vi "Standard Engine.vi"(8 "error in":errorcluster, 11 "Engine Process Init Data":T1) -> (0 "error out":errorcluster)   [LabVIEW 2013, in "Standard Engine Runtime.lvclass"]
doc: "This VI is a process that executes modules and has an API for transitioning through its state machine. Once it is initialized and running, it calls an array of module input methods, followed by an array of module process methods, followed by an array of module output methods, and then does any necessary error handling and bookkeeping."
uses:
  Standard Engine Runtime.lvclass
  Engine Process Init Data.ctl
  Commands.ctl
  Engine Config Data.ctl
  Configuration/Standard Engine Configuration.lvclass
  <vilib>/NI/Tag Bus Module Framework/runtime/TBM module execution interface.lvclass
  <vilib>/NI/Tag Bus Module Framework/module configuration/TBM module configuration.lvclass
  <vilib>/NI/Module Execution Interface/Engine Runtime/Execution States.ctl
  Engine Data.ctl
  Configuration/Loop Info.ctl
  <vilib>/NI/Tag Bus/table/data table.ctl
  Module Execution Info.ctl
  Data Table with Transfer Spec.ctl
  <vilib>/NI/Tag Bus/table/transfer specification.ctl
  <vilib>/NI/Tag Bus/tag/Data Type.ctl
  Configuration/Module Decimation.ctl
  Configuration/Module Error Configuration.ctl
  Configuration/Error Actions By Category.ctl
  <vilib>/NI/Tag Bus Module Framework/runtime/error classification.ctl
  Configuration/Error Actions.ctl
  <vilib>/NI/Module Timing Source/timing source/TBM timing source.lvclass
  Configuration/timing policy.ctl
  async execution info.ctl
  asynchronous process data.ctl
  async command notification.ctl
  <vilib>/NI/Tag Bus Module Framework/runtime/execution settings.ctl
  async error info.ctl
  status reporting data.ctl
  module status reporting.ctl
  <vilib>/Platform/TimedLoop/XDataNode/timing_clust.ctl
  <vilib>/Platform/TimedLoop/XDataNode/nitl_modes.ctl
  <vilib>/Platform/TimedLoop/XDataNode/wakeup.ctl
  <vilib>/NI/Module Timing Source/timing source/TBM timing source.lvclass/TBM timing source.ctl
  <vilib>/NI/Tag Bus/table/transfer table data.vi
  Module Execution Decimation.vi
  Error Handler.vi
  <vilib>/NI/Tag Bus/table/write data element.vi
  <vilib>/NI/Tag Bus/table/data polymorphs/write one/write Boolean.vi
  <vilib>/NI/Tag Bus/table/data polymorphs/write one/write U32.vi
  <vilib>/NI/Tag Bus/table/data polymorphs/write one/write U64.vi
  <vilib>/NI/Tag Bus/table/data polymorphs/write one/write I32.vi
  Delete Module Index.vi
  <vilib>/platform/TimedLoop/XDataNode/XDataNode.xnode
  <vilib>/NI/Module Execution Interface/Engine Runtime/Engine Runtime Interface.lvclass
  <vilib>/NI/Tag Bus/table/data table.lvlib
  <vilib>/NI/Tag Bus/tag/tag descriptor.lvclass
  <vilib>/Platform/TimedLoop/XDataNode/XDNodeRunTimeDep.lvlib
panel:
  out "iterations":i32
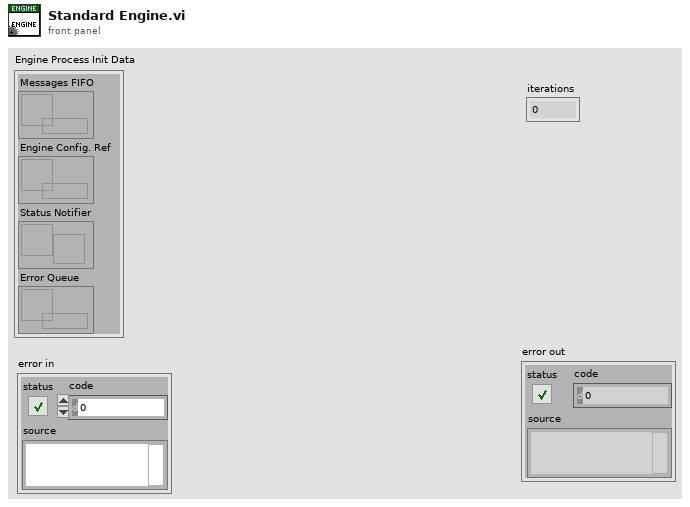
[diagram p1: front panel]
types:
  T1 = typedef "Standard Engine Runtime.lvclass/Engine Process Init Data.ctl" = cluster{"Messages FIFO":refnum<k33>, "Engine Config. Ref":refnum<data-value>, "Status Notifier":refnum<notifier>, "Error Queue":refnum<queue>}
  T2 = typedef "Standard Engine Runtime.lvclass/Engine Data.ctl" = cluster{"Loop Info":T3, "Main Tag Data":T4, "Module Info":T5, "engine timing source":refnum<class "TBM timing source.lvclass">, "timing policy":T14, "async execution info":T15, "status reporting":T18}
  T3 = typedef "Standard Engine Configuration.lvclass/Loop Info.ctl" = cluster{"Processor":i32, "Priority":i32}
  T4 = typedef "tag bus.lvlib/data table.lvlib/data table.ctl" = cluster{"Double":dbl[], "Single":sgl[], "I64":i64[], "I32":i32[], "I16":i16[], "I8":i8[], "U64":u64[], "U32":u32[], "U16":u16[], "U8":u8[], "Boolean":bool[], "String":string[], "Array of Double":cluster{"DBL Array":dbl[]}[], "Array of Single":cluster{"SGL Array":sgl[]}[], "Array of I64":cluster{"I64 Array":i64[]}[], "Array of I32":cluster{"I32 Array":i32[]}[], "Array of I16":cluster{"I16 Array":i16[]}[], "Array of I8":cluster{"I8 Array":i8[]}[], "Array of U64":cluster{"U64 Array":u64[]}[], "Array of U32":cluster{"U32 Array":u32[]}[], "Array of U16":cluster{"U16 Array":u16[]}[], "Array of U8":cluster{"U8 Array":u8[]}[], "Array of Boolean":cluster{"Boolean Array":bool[]}[], "Array of String":cluster{"String Array":string[]}[]}
  T5 = typedef "Standard Engine Runtime.lvclass/Module Execution Info.ctl" = cluster{"Tag Bus Modules":refnum<class "TBM module execution interface.lvclass">[], "Execute?":bool[], "Input Method Indices":i32[], "Process Method Indices":i32[], "Output Method Indices":i32[], "Input Transfer Specifications":T6[], "Parameter Transfer Specifications":T6[], "Result Transfer Specifications":T6[], "Output Transfer Specifications":T6[], "Module Errors":errorcluster[], "Module Decimation":T9[], "Module Decimation Indices":i32[], "Error Queue":refnum<queue>, "Module Error Configuration":T10[], "Module Errors (n-1)":errorcluster[]}
  T6 = typedef "Standard Engine Runtime.lvclass/Data Table with Transfer Spec.ctl" = cluster{"Data Table":T4, "Transfer Specification":T7[]}
  T7 = typedef "tag bus.lvlib/data table.lvlib/transfer specification.ctl" = cluster{"data type":T8, "sink indices":i32[], "source indices":i32[]}
  T8 = typedef "tag bus.lvlib/tag descriptor.lvclass/Data Type.ctl" = enum16{"Double", "Single", "I64", "I32", "I16", "I8", "U64", "U32", "U16", "U8", "Boolean", "String", "Array of Double", "Array of Single", "Array of I64", "Array of I32", "Array of I16", "Array of I8", "Array of U64", "Array of U32", "Array of U16", "Array of U8", "Array of Boolean", "Array of String"}
  T9 = typedef "Standard Engine Configuration.lvclass/Module Decimation.ctl" = cluster{"Decimation":u16, "Offset":u16}
  T10 = typedef "Standard Engine Configuration.lvclass/Module Error Configuration.ctl" = cluster{"Module Error Configuration":T11[]}
  T11 = typedef "Standard Engine Configuration.lvclass/Error Actions By Category.ctl" = cluster{"error classification":T12, "Error Actions":T13[]}
  T12 = typedef "TBM module execution interface.lvclass/error classification.ctl" = enum16{"unknown", "none", "trivial", "recoverable", "critical"}
  T13 = typedef "Standard Engine Configuration.lvclass/Error Actions.ctl" = enum16{"Clear", "Notify", "Stop Component", "Stop Engine", "Safe State", "Attempt Recovery"}
  T14 = typedef "Standard Engine Configuration.lvclass/timing policy.ctl" = enum16{"strict determinism", "nonblocking", "nondeterministic inline"}
  T15 = typedef "Standard Engine Runtime.lvclass/async execution info.ctl" = cluster{"Tag Bus Modules":T16[], "Execute?":bool[], "Input Method Indices":i32[], "Process Method Indices":i32[], "Output Method Indices":i32[], "Input Transfer Specifications":T6[], "Parameter Transfer Specifications":T6[], "Result Transfer Specifications":T6[], "Output Transfer Specifications":T6[], "Module Errors":errorcluster[], "Module Decimation":T9[], "Module Decimation Indices":i32[], "Error Queue":refnum<queue>, "Module Error Configuration":T10[], "comm errors":errorcluster[]}
  T16 = typedef "Standard Engine Runtime.lvclass/asynchronous process data.ctl" = cluster{"thread reference":refnum<vi>, "cmd notification":refnum<k33>, "execution period (ms)":i32, "input from component":refnum<queue>, "input to component":refnum<queue>, "output from component":refnum<queue>, "output to component":refnum<queue>, "process input from component":refnum<queue>, "process input to component":refnum<queue>, "process result from component":refnum<queue>, "process result to component":refnum<queue>, "execution settings":T17, "error fifo":refnum<k33>}
  T17 = typedef "TBM module execution interface.lvclass/execution settings.ctl" = cluster{"reads inputs":bool, "processes data":bool, "writes outputs":bool}
  T18 = typedef "Standard Engine Runtime.lvclass/status reporting data.ctl" = cluster{"late index (bool)":i32, "late count (U32)":i32, "current dt ns(U64)":i32, "synchronous modules":T19[], "asynchronous modules":T19[]}
  T19 = typedef "Standard Engine Runtime.lvclass/module status reporting.ctl" = cluster{"module index":i32, "error tag (I32)":i32}
  T20 = typedef "Engine Runtime Interface.lvclass/Execution States.ctl" = enum16{"Initializing", "Paused (Initialized)", "Running", "Set Safe Outputs", "Uninitializing", "Stopped (Uninitialized)", "Error (Uninitialized)", "Safe State (Uninitialized)", "Closed"}
  T21 = typedef "Standard Engine Runtime.lvclass/Commands.ctl" = enum16{"Initialize", "Start", "Pause", "Safe State", "Normal", "Stop", "Shutdown"}
  T22 = typedef "XDNodeRunTimeDep.lvlib/timing_clust.ctl" = cluster{"Expected End [f-1]":u64, "Actual End [f-1]":u64, "Finished Late? [f-1]":bool, "Expected End [i-1]":u64, "Actual End [i-1]":u64, "Finished Late? [i-1]":bool, "Expected Start [i]":u64, "Actual Start [i]":u64, "Expected Start [f]":u64, "Actual Start [f]":u64, "Source Name":string, "Structure Name":string, "Period":i64, "Deadline":i64, "Offset":i64, "Start":i64, "Priority":i32, "Timeout":i32, "Mode":T23, "Wakeup Reason":T24, "Error":errorcluster, "Source Type":string, "Secondary Source Type":string, "Global End Time":u64, "Global Start Time":u64, "Frame Duration":u64, "Iteration Duration":u64, "Assigned CPU":i32, "I/O Scan Engine Mode":u32}
  T23 = typedef "XDNodeRunTimeDep.lvlib/nitl_modes.ctl" = enum32{"No Change", "Process missed periods, maintain original phase", "Discard missed periods, maintain original phase", "Process missed periods, ignore original phase", "Discard missed periods, ignore original phase"}
  T24 = typedef "XDNodeRunTimeDep.lvlib/wakeup.ctl" = enum32{"Normal", "Aborted", "Asynchronous wakeup", "Timing source error", "Timed loop error", "Timeout"}
  T25 = typedef "Standard Engine Runtime.lvclass/Engine Config Data.ctl" = cluster{"Engine Configuration":refnum<class "Standard Engine Configuration.lvclass">, "Modules":refnum<class "TBM module execution interface.lvclass">[], "Module Configurations":refnum<class "TBM module configuration.lvclass">[]}
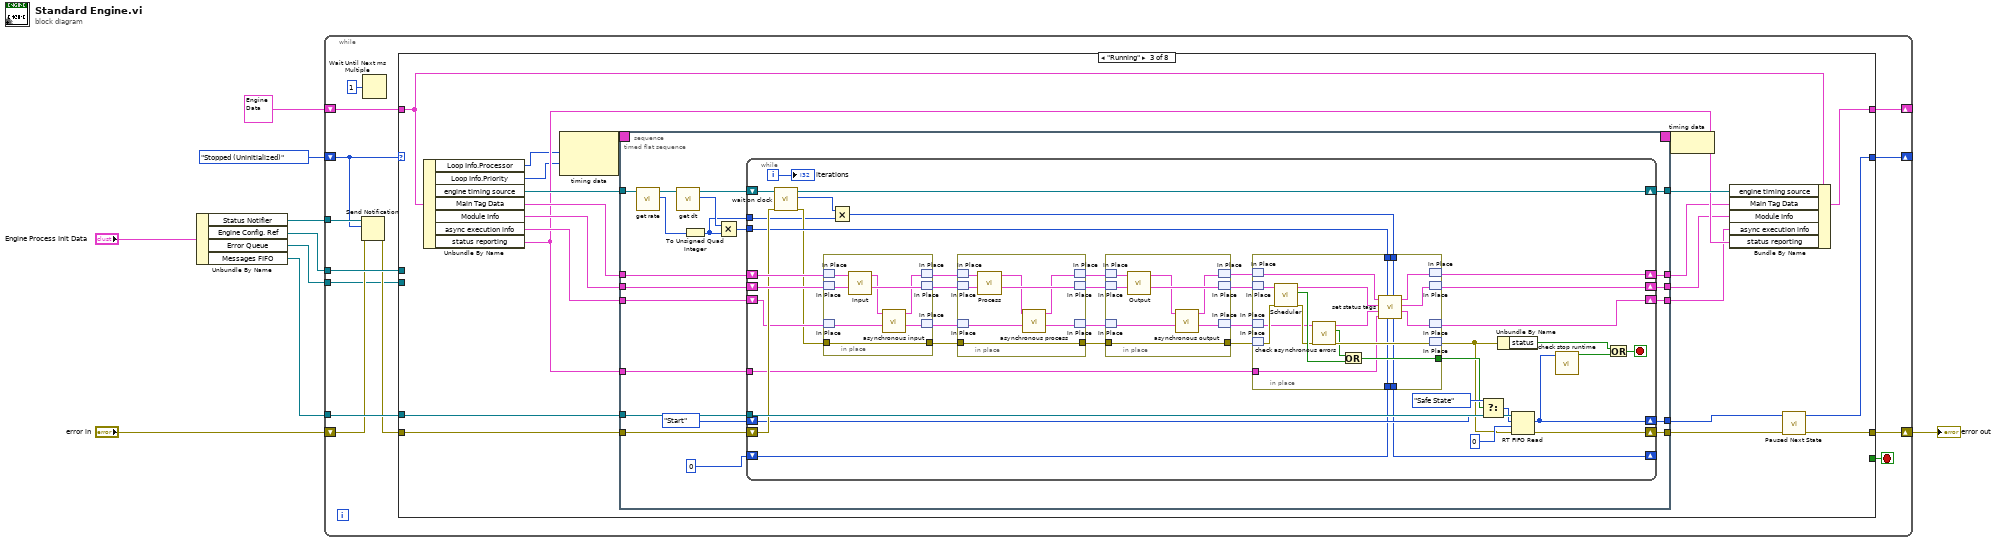
[diagram p0: block diagram]
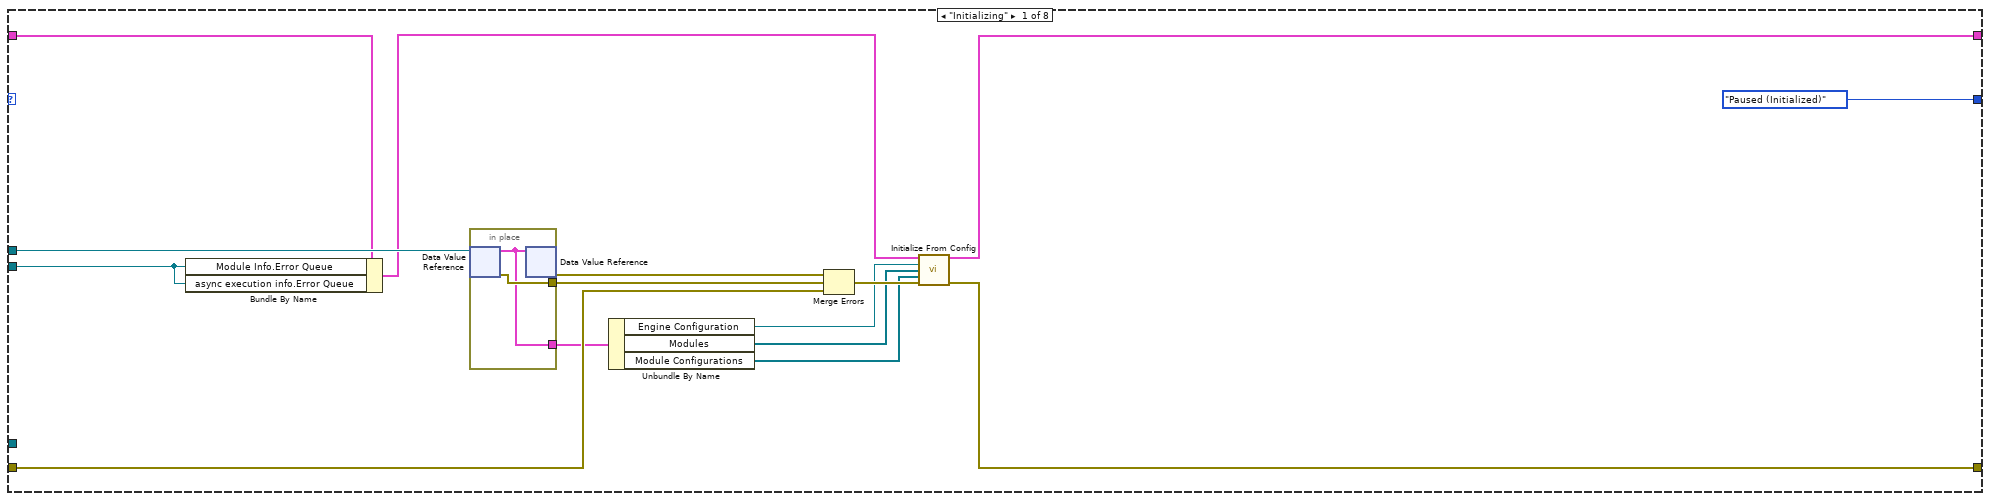
[diagram p2: hidden frame]
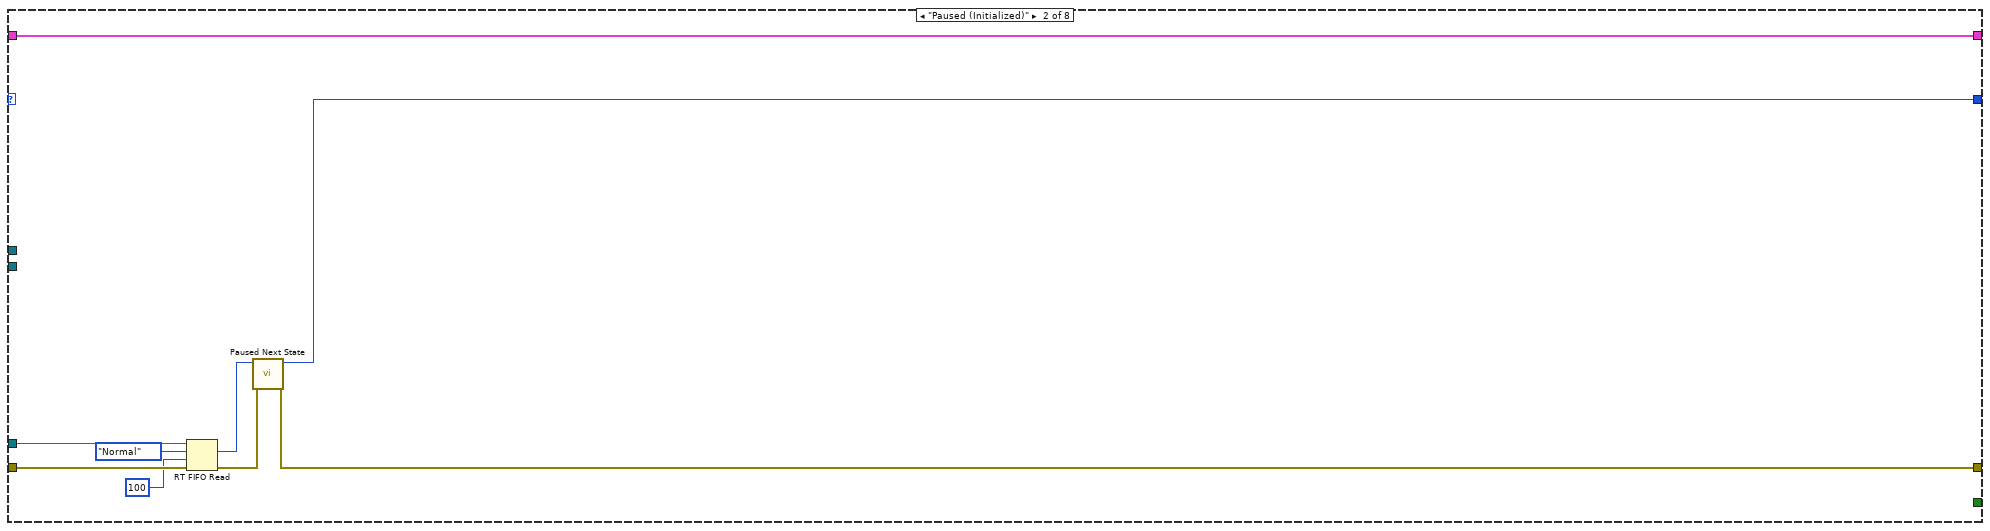
[diagram p3: hidden frame]
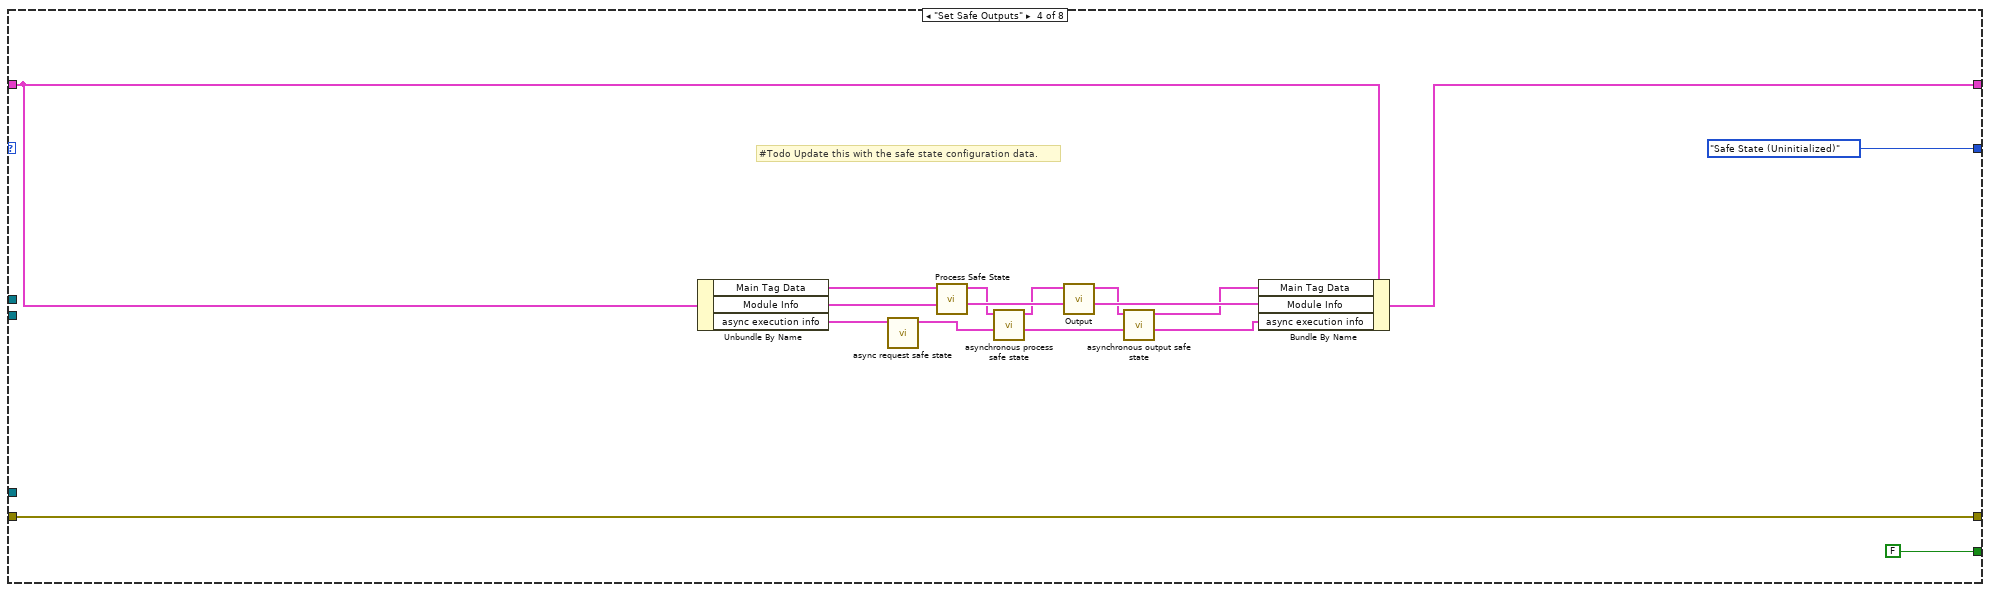
[diagram p4: hidden frame]
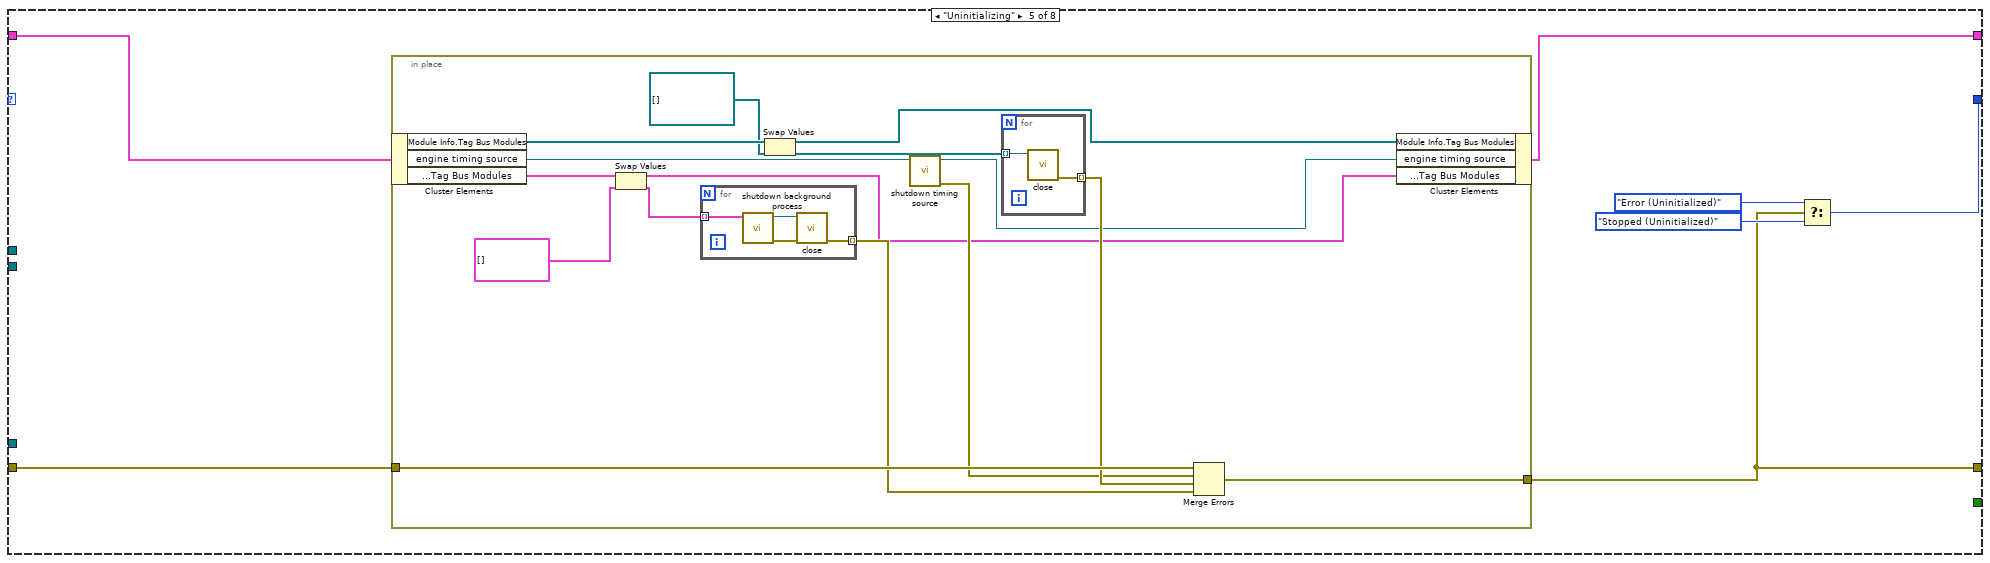
[diagram p5: hidden frame]
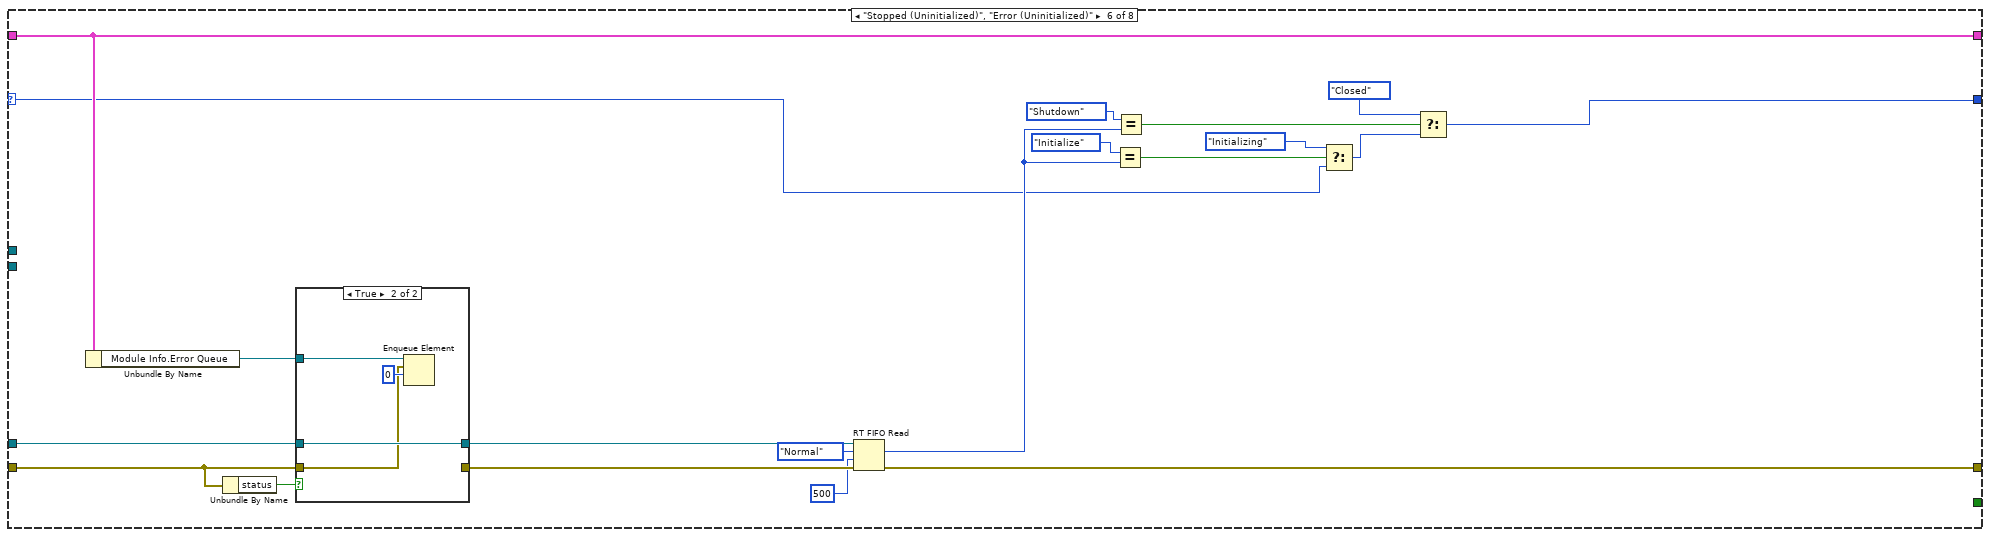
[diagram p6: hidden frame]
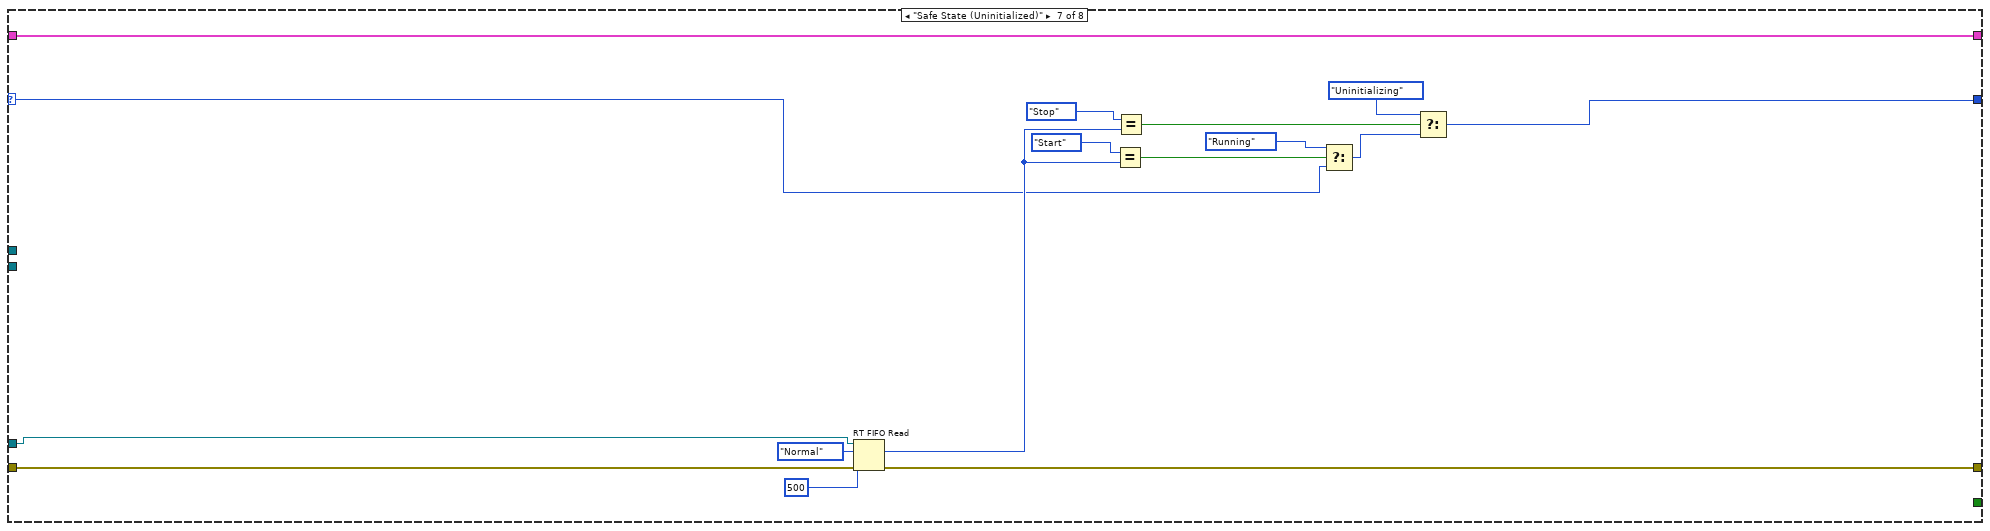
[diagram p8: hidden frame]
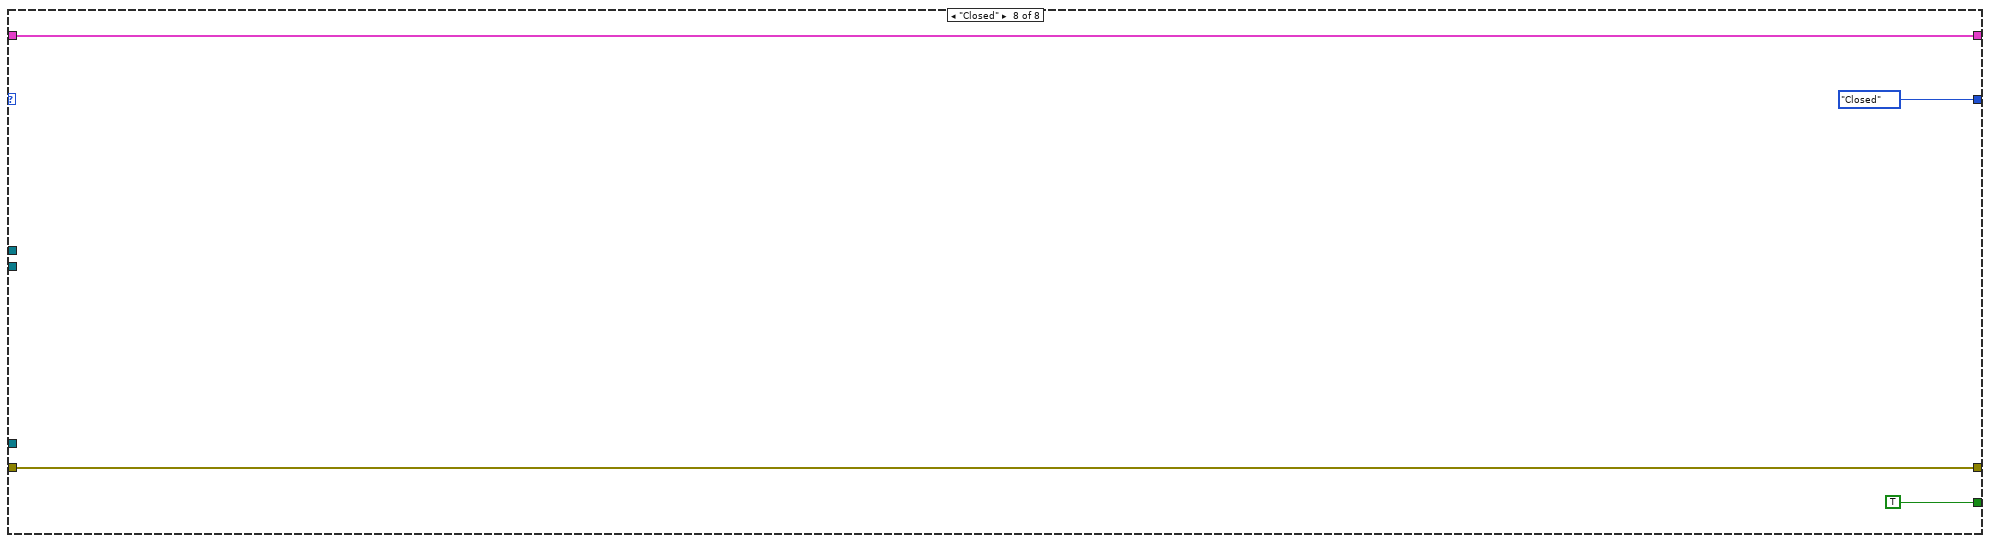
[diagram p9: hidden frame]
diagram:
  n1 = Unbundle By Name("Engine Process Init Data") -> ("Status Notifier"=w7:refnum<notifier>, "Engine Config. Ref"=w6:refnum<data-value>, "Error Queue"=w3:refnum<queue>, "Messages FIFO"=w5:refnum<k33>)
  n2 = while {
    shift-right: [w19] -> _
    shift-left: Execution_States."Stopped (Uninitialized)" ("States") -> [w14]
    shift-right: [w20] -> _
    shift-left: T2 {"Loop Info"={"Processor"=-2, "Priority"=0}, "Main Tag Data"={"Double"=[], "Single"=[], "I64"=[], "I32"=[], "I16"=[], "I8"=[], "U64"=[], "U32"=[], "U16"=[], "U8"=[], "Boolean"=[], "String"=[], "Array of Double"=[], "Array of Single"=[], "Array of I64"=[], "Array of I32"=[], "Array of I16"=[], "Array of I8"=[], "Array of U64"=[], "Array of U32"=[], "Array of U16"=[], "Array of U8"=[], "Array of Boolean"=[], "Array of String"=[]}, "Module Info"={"Tag Bus Modules"=[], "Execute?"=[], "Input Method Indices"=[], "Process Method Indices"=[], "Output Method Indices"=[], "Input Transfer Specifications"=[], "Parameter Transfer Specifications"=[], "Result Transfer Specifications"=[], "Output Transfer Specifications"=[], "Module Errors"=[], "Module Decimation"=[], "Module Decimation Indices"=[], "Error Queue"=refnum, "Module Error Configuration"=[], "Module Errors (n-1)"=[]}, "engine timing source"=refnum, "timing policy"=enum."nonblocking", "async execution info"={"Tag Bus Modules"=[], "Execute?"=[], "Input Method Indices"=[], "Process Method Indices"=[], "Output Method Indices"=[], "Input Transfer Specifications"=[], "Parameter Transfer Specifications"=[], "Result Transfer Specifications"=[], "Output Transfer Specifications"=[], "Module Errors"=[], "Module Decimation"=[], "Module Decimation Indices"=[], "Error Queue"=refnum, "Module Error Configuration"=[], "comm errors"=[]}, "status reporting"={"late index (bool)"=0, "late count (U32)"=0, "current dt ns(U64)"=0, "synchronous modules"=[], "asynchronous modules"=[]}} ("Engine Data Out") -> [w22]
    shift-right: [w21] -> w8
    shift-left: "error in" -> [w13]
    tunnel: w5 -> [w18]
    tunnel: w6 -> [w16]
    tunnel: w7 -> [w15]
    tunnel: w3 -> [w11]
    stop <- w17 stop-if-true
    n3 = Send Notification(notification=w14, notifier=w15, error in (no error)=w13) -> (error out=w12:errorcluster)  [unwired: 1 out]
    n4 = Wait Until Next ms Multiple(millisecond multiple=u32 1) -> ()  [unwired: 1 out]
    n5 = case shown="\"Running\"" w14 {
      selector: w14 -> [_ _ _ _ _ w245 w269 _]
      tunnel: w22 -> [w26 w48 w67 w208 w214 w247 w270 w284]
      tunnel: w12 -> [w34 w47 w53 w212 w216 w241 w272 w286]
      tunnel: [w24 w42 w65 w212 w215 w256 w279 w286] -> w21
      tunnel: [w32 w48 w66 w209 w213 w247 w270 w284] -> w20
      tunnel: [Execution_States."Paused (Initialized)" ("States") w46 w68 Execution_States."Safe State (Uninitialized)" ("States") w217 w257 w280 Execution_States."Closed" ("States")] -> w19
      tunnel: w18 -> [_ w41 w69 _ _ w249 w271 _]
      tunnel: [_ _ _ FALSE _ _ _ TRUE] -> w17
      tunnel: w16 -> [w29 _ _ _ _ _ _ _]
      tunnel: w11 -> [w23 _ _ _ _ _ _ _]
      frame "Initializing" {
        n6 = Bundle By Name(cluster=w26, "Module Info.Error Queue"=w23, "async execution info.Error Queue"=w23) -> (w25:T2)
        n7 = in-place {
          in-place-border: [w39] -> w35
          in-place-border: [w38] -> w33
          n8 = in-place-dvr #1(w29) -> (w38:T25, w39:errorcluster)
          n9 = in-place-dvr #1(w38) -> (w36:errorcluster)  [unwired: 1 out]
        }
        n10 = Unbundle By Name(w33) -> ("Engine Configuration"=w30:refnum<class "Standard Engine Configuration.lvclass">, "Modules"=w28:refnum<class "TBM module execution interface.lvclass">[], "Module Configurations"=w27:refnum<class "TBM module configuration.lvclass">[])
        n11 = Merge Errors(w36, w35, w34) -> (w31:errorcluster)
        n12 = call "Initialize From Config.vi"("Engine Data"=w25, "Engine Configuration"=w30, "Modules"=w28, "Module Configurations"=w27, "error in"=w31) -> ("Engine Data Out"=w32:T2, "error out"=w24:errorcluster)  [unwired: 9 in]
      }
      frame "Paused (Initialized)" {
        n13 = RT FIFO Read(0:w41, 1:Commands."Normal" ("Commands"), 2:100 ("timeout in ms (0)"), 3:w47) -> (9:w45:T21, 11:w44:errorcluster)  [unwired: 3 out]
        n14 = call "Paused Next State.vi"("error in"=w44, "Command"=w45) -> ("error out"=w42:errorcluster, "State"=w46:T20)  [unwired: 8 in]
      }
      frame "Running" {
        n15 = Unbundle By Name(w67) -> ("Loop Info.Processor"=w50:i32, "Loop Info.Priority"=w49:i32, "engine timing source"=w62:refnum<class "TBM timing source.lvclass">, "Main Tag Data"=w61:T4, "Module Info"=w60:T5, "async execution info"=w59:T15, "status reporting"=w57:T18)
        n16 = node-c288(w50, w49) -> (w52:T22)
        n17 = timed-sequence {
          timing: w52 -> [_]
          timing-out: [_] -> w51
          tunnel: w69 -> [w82]
          tunnel: [w81] -> w64
          tunnel: [w80] -> w63
          tunnel: w62 -> [w70]
          tunnel: w61 -> [w79]
          tunnel: w60 -> [w78]
          tunnel: w59 -> [w77]
          tunnel: [w76] -> w58
          tunnel: w57 -> [w75]
          tunnel: [w74] -> w56
          tunnel: [w73] -> w55
          tunnel: [w72] -> w54
          tunnel: w53 -> [w71]
          n18 = timed-flat-sequence {
            tunnel: w82 -> [w103]
            tunnel: [w102] -> w81
            tunnel: [w101] -> w80
            tunnel: w79 -> [w100]
            tunnel: w78 -> [w99]
            tunnel: w77 -> [w98]
            tunnel: [w97] -> w76
            tunnel: w75 -> [w96]
            tunnel: [w95] -> w74
            tunnel: [w94] -> w73
            tunnel: [w93] -> w72
            tunnel: w71 -> [w89]
            tunnel: w70 -> [w88]
            n19 = call-dynamic "get rate.vi"("timing source in"=w88) -> ("period (ns)"=w84:i64, "timing source out"=w87:refnum<class "TBM timing source.lvclass">)  [unwired: 8 in, 1 out]
            n20 = call <vilib>:"get dt.vi"("timing source in"=w87) -> ("dt"=w85:u32, "timing source out"=w91:refnum<class "TBM timing source.lvclass">)  [unwired: 9 in]
            n21 = To Unsigned Quad Integer(1:w84) -> (0:w83:u64)
            n22 = Multiply(x=w85, y=w83) -> (x*y=w86:u64)
            n23 = while {
              tunnel: w103 -> [w135]
              shift-right: [w137] -> w102
              shift-left: Commands."Start" ("Commands") -> [w123]
              shift-right: [w117] -> w95
              shift-left: w100 -> [w144]
              shift-right: [w138] -> w94
              shift-left: w99 -> [w143]
              shift-right: [w134] -> w101
              shift-left: w89 -> [w130]
              shift-right: [w129] -> w97
              shift-left: w91 -> [w131]
              tunnel: w86 -> [w116]
              shift-right: [w124] -> w93
              shift-left: w98 -> [w128]
              tunnel: w96 -> [w115]
              shift-right: [w114] -> _
              shift-left: u32 0 ("late count out") -> [w113]
              tunnel: w83 -> [w108]
              i -> [w133]
              stop <- w105 stop-if-true
              n24 = call-dynamic "wait on clock.vi"("error in"=w130, "timing source in"=w131) -> ("error out"=w112:errorcluster, "ticks since last call"=w107:u32, "timing source out"=w129:refnum<class "TBM timing source.lvclass">)  [unwired: 7 in]
              n25 = in-place {
                in-place-border: w112 -> [w184]
                in-place-border: [w184] -> w109
                n26 = in-place-match #2(w144) -> (w183:T4)
                n27 = in-place-match #3(w143) -> (w188:T5)
                n28 = in-place-match #4(w128) -> (w186:T15)
                n29 = call "Input.vi"("Module Info In"=w188, "Engine Tags In"=w183) -> ("Module Info Out"=w187:T5, "Engine Tags Out"=w182:T4)  [unwired: 8 in]
                n30 = call "asynchronous input.vi"("Module Info In"=w186, "Engine Tags In"=w182) -> ("Module Info Out"=w185:T15, "Engine Tags Out"=w181:T4)  [unwired: 8 in]
                n31 = in-place-match #2(w181) -> (w142:T4)
                n32 = in-place-match #3(w187) -> (w141:T5)
                n33 = in-place-match #4(w185) -> (w127:T15)
              }
              n34 = Multiply(x=w107, y=w108) -> (x*y=w106:u64)
              n35 = in-place {
                in-place-border: [w173] -> w110
                in-place-border: w109 -> [w173]
                n36 = in-place-match #5(w142) -> (w179:T4)
                n37 = in-place-match #6(w141) -> (w180:T5)
                n38 = in-place-match #7(w127) -> (w177:T15)
                n39 = call "Process.vi"("Module Info In"=w180, "Engine Tags In"=w179) -> ("Module Info Out"=w178:T5, "Engine Tags Out"=w176:T4)  [unwired: 8 in]
                n40 = call "asynchronous process.vi"("Module Info In"=w177, "Engine Tags In"=w176) -> ("Module Info Out"=w175:T15, "Engine Tags Out"=w174:T4)  [unwired: 8 in]
                n41 = in-place-match #5(w174) -> (w132:T4)
                n42 = in-place-match #6(w178) -> (w140:T5)
                n43 = in-place-match #7(w175) -> (w126:T15)
              }
              n44 = in-place {
                in-place-border: [w165] -> w111
                in-place-border: w110 -> [w165]
                n45 = in-place-match #8(w132) -> (w172:T4)
                n46 = in-place-match #9(w140) -> (w171:T5)
                n47 = in-place-match #10(w126) -> (w169:T15)
                n48 = call "Output.vi"("Module Info In"=w171, "Engine Tags In"=w172) -> ("Module Info Out"=w170:T5, "Engine Tags Out"=w167:T4)  [unwired: 8 in]
                n49 = call "asynchronous output.vi"("Module Info In"=w169, "Engine Tags In"=w167) -> ("Module Info Out"=w168:T15, "Engine Tags Out"=w166:T4)  [unwired: 8 in]
                n50 = in-place-match #8(w166) -> (w118:T4)
                n51 = in-place-match #9(w170) -> (w139:T5)
                n52 = in-place-match #10(w168) -> (w125:T15)
              }
              n53 = in-place {
                in-place-border: [w160] -> w120
                in-place-border: w116 -> [w147]
                in-place-border: w106 -> [w146]
                in-place-border: w115 -> [w148]
                in-place-border: [w150] -> w114
                in-place-border: w113 -> [w149]
                n54 = in-place-match #11(w118) -> (w156:T4)
                n55 = in-place-match #12(w139) -> (w157:T5)
                n56 = in-place-match #13(w125) -> (w158:T15)
                n57 = in-place-match #14(w111) -> (w164:errorcluster)
                n58 = call "Scheduler.vi"("error in"=w164, "Module Info In"=w157) -> ("error out"=w162:errorcluster, "Safe State?"=w163:bool, "Module Info Out"=w155:T5)  [unwired: 7 in]
                n59 = call "check asynchronous errors.vi"("error in"=w162, "Module Info In"=w158) -> ("error out"=w161:errorcluster, "safe state?"=w159:bool, "Module Info Out"=w152:T15)  [unwired: 7 in]
                n60 = Or(x=w159, y=w163) -> (x .or. y?=w160:bool)
                n61 = call "set status tags.vi"("ns since last call"=w146, "late count in"=w149, "desired dt ns"=w147, "status reporting"=w148, "async module info in"=w152, "Module Info In"=w155, "Engine Tags In"=w156) -> ("async module info out"=w151:T15, "Module Info Out"=w153:T5, "Engine Tags Out"=w154:T4, "late count out"=w150:u32)  [unwired: 1 in]
                n62 = in-place-match #11(w154) -> (w117:T4)
                n63 = in-place-match #12(w153) -> (w138:T5)
                n64 = in-place-match #13(w151) -> (w124:T15)
                n65 = in-place-match #14(w161) -> (w119:errorcluster)
              }
              n66 = Select(t=Commands."Safe State" ("y"), s=w120, f=w123) -> (s? t:f=w122:T21)
              n67 = Unbundle By Name(w119) -> ("status"=w104:bool)
              n68 = RT FIFO Read(0:w135, 1:w122, 2:0 ("timeout in ms (0)"), 3:w119) -> (9:w137:T21, 11:w134:errorcluster)  [unwired: 3 out]
              n69 = call "check stop runtime.vi"("Commands"=w137) -> ("stop?"=w136:bool)  [unwired: 10 in]
              n70 = Or(x=w104, y=w136) -> (x .or. y?=w105:bool)
              "iterations" <- w133
            }
          }
        }
        n71 = node-c288(w51) -> ()
        n72 = Bundle By Name(cluster=w67, "engine timing source"=w58, "Main Tag Data"=w56, "Module Info"=w55, "async execution info"=w54, "status reporting"=w57) -> (w66:T2)
        n73 = call "Paused Next State.vi"("error in"=w63, "Command"=w64) -> ("error out"=w65:errorcluster, "State"=w68:T20)  [unwired: 8 in]
      }
      frame "Set Safe Outputs" {
        # "#Todo Update this with the safe state configuration data."
        n74 = Unbundle By Name(w208) -> ("Main Tag Data"=w207:T4, "Module Info"=w206:T5, "async execution info"=w200:T15)
        n75 = call "async request safe state.vi"("async execution info in"=w200) -> ("async execution info out"=w201:T15)  [unwired: 10 in]
        n76 = call "Process Safe State.vi"("Module Info In"=w206, "Engine Tags In"=w207) -> ("Module Info Out"=w205:T5, "Engine Tags Out"=w203:T4)  [unwired: 8 in]
        n77 = call "asynchronous process safe state.vi"("Module Info In"=w201, "Engine Tags In"=w203) -> ("Module Info Out"=w196:T15, "Engine Tags Out"=w202:T4)  [unwired: 8 in]
        n78 = call "Output.vi"("Module Info In"=w205, "Engine Tags In"=w202) -> ("Module Info Out"=w204:T5, "Engine Tags Out"=w199:T4)  [unwired: 8 in]
        n79 = call "asynchronous output safe state.vi"("Module Info In"=w196, "Engine Tags In"=w199) -> ("Module Info Out"=w197:T15, "Engine Tags Out"=w198:T4)  [unwired: 8 in]
        n80 = Bundle By Name(cluster=w208, "Main Tag Data"=w198, "Module Info"=w204, "async execution info"=w197) -> (w209:T2)
      }
      frame "Uninitializing" {
        n81 = in-place {
          in-place-border: w216 -> [w234]
          in-place-border: [w233] -> w215
          n82 = in-place-cluster #15(w214) -> ("Module Info.Tag Bus Modules"=w223:refnum<class "TBM module execution interface.lvclass">[], "engine timing source"=w229:refnum<class "TBM timing source.lvclass">, "async execution info.Tag Bus Modules"=w228:T16[])
          n83 = Swap Values(12:w228, 14:T16[] []) -> (1:w225:T16[], 3:w227:T16[])  [unwired: 1 in]
          n84 = for {
            tunnel: [w236] -> w230 mode=indexing
            tunnel: w227 -> [w235] mode=indexing
            n85 = call "shutdown background process.vi"("async data"=w235) -> ("error out"=w238:errorcluster, "module out"=w237:refnum<class "TBM module execution interface.lvclass">)  [unwired: 8 in, 1 out]
            n86 = call-dynamic "close.vi"("error in"=w238, "module in"=w237) -> ("error out"=w236:errorcluster)  [unwired: 9 in]
          }
          n87 = Swap Values(12:w223, 14:refnum<class "TBM module execution interface.lvclass">[] [] ("y'")) -> (1:w221:refnum<class "TBM module execution interface.lvclass">[], 3:w222:refnum<class "TBM module execution interface.lvclass">[])  [unwired: 1 in]
          n88 = call-dynamic "shutdown timing source.vi"("timing source in"=w229) -> ("error out"=w231:errorcluster, "timing source out"=w224:refnum<class "TBM timing source.lvclass">)  [unwired: 9 in]
          n89 = for {
            tunnel: w222 -> [w240] mode=indexing
            tunnel: [w239] -> w232 mode=indexing
            n90 = call-dynamic "close.vi"("module in"=w240) -> ("error out"=w239:errorcluster)  [unwired: 10 in]
          }
          n91 = Merge Errors(w234, w231, w232, w230) -> (w233:errorcluster)
          n92 = in-place-cluster #15("Module Info.Tag Bus Modules"=w221, "engine timing source"=w224, "async execution info.Tag Bus Modules"=w225) -> (w213:T2)
        }
        n93 = Select(t=Execution_States."Error (Uninitialized)" ("States"), s=w215, f=Execution_States."Stopped (Uninitialized)" ("States")) -> (s? t:f=w217:T20)
      }
      frame "Stopped (Uninitialized)", "Error (Uninitialized)" {
        n94 = Unbundle By Name(w247) -> ("Module Info.Error Queue"=w246:refnum<queue>)
        n95 = Unbundle By Name(w241) -> ("status"=w242:bool)
        n96 = case shown="True" w242 {
          tunnel: w249 -> [w262 w266]
          tunnel: [w262 w266] -> w248
          tunnel: [w261 _] -> w244
          tunnel: w246 -> [_ w265]
          tunnel: w241 -> [w261 w263]
          frame False {
          }
          frame True {
            n97 = Enqueue Element(queue=w265, element=w263, timeout in ms (-1)=0) -> ()  [unwired: 1 in, 3 out]
          }
        }
        n98 = RT FIFO Read(0:w248, 1:Commands."Normal" ("Commands"), 2:500 ("milliseconds to wait"), 3:w244) -> (9:w260:T21, 11:w256:errorcluster)  [unwired: 3 out]
        n99 = Equal?(x=Commands."Initialize" ("Commands"), y=w260) -> (x = y?=w259:bool)
        n100 = Equal?(x=Commands."Shutdown" ("Commands"), y=w260) -> (x = y?=w255:bool)
        n101 = Select(t=Execution_States."Initializing" ("States"), s=w259, f=w245) -> (s? t:f=w258:T20)
        n102 = Select(t=Execution_States."Closed" ("States"), s=w255, f=w258) -> (s? t:f=w257:T20)
      }
      frame "Safe State (Uninitialized)" {
        n103 = RT FIFO Read(0:w271, 1:Commands."Normal" ("Commands"), 2:500 ("timeout in ms (0)"), 3:w272) -> (9:w282:T21, 11:w279:errorcluster)  [unwired: 3 out]
        n104 = Equal?(x=Commands."Start" ("Commands"), y=w282) -> (x = y?=w267:bool)
        n105 = Equal?(x=Commands."Stop" ("Commands"), y=w282) -> (x = y?=w278:bool)
        n106 = Select(t=Execution_States."Running" ("States"), s=w267, f=w269) -> (s? t:f=w281:T20)
        n107 = Select(t=Execution_States."Uninitializing" ("States"), s=w278, f=w281) -> (s? t:f=w280:T20)
      }
      frame "Closed" {
      }
    }
  }
  "error out" <- w8
